vi "SendCmdToSkywireWaitToken.vi"(5 "Flush after? (y)":bool, 6 "Timeout (mSecs)":dbl=3500.0, 7 "Display err mess?":bool=TRUE, 8 "error in (no error)":errorcluster, 9 "Wait for token":string, 10 "Cmd String":string="AT+CSQ", 11 "VISA resource name":refnum<visa-resource-name>="COM30") -> (0 "error out":errorcluster, 1 "Response":string, 2 "timeout":bool, 3 "VISA resource name out":refnum<visa-resource-name>="COM30", 4 "Log resp":string)   [LabVIEW 2013]
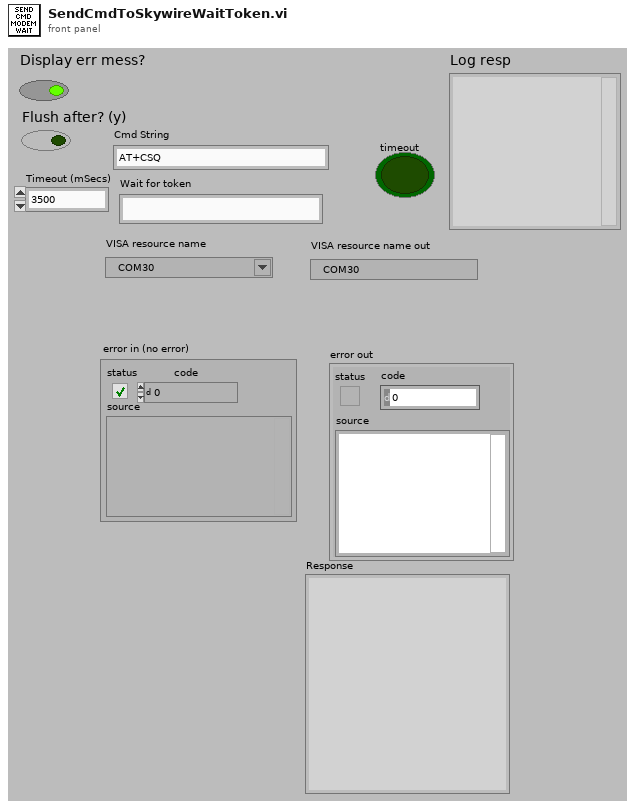
[diagram p1: front panel]
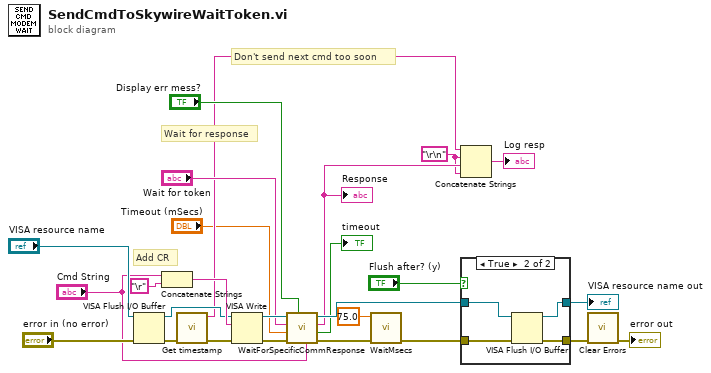
[diagram p0: block diagram]
diagram:
  w4 = "\r\n"
  # "Don't send next cmd too soon"
  # "Wait for response"
  # "Add CR"
  n1 = VISA Flush I/O Buffer(VISA resource name="VISA resource name", error in (no error)="error in (no error)") -> (VISA resource name out=w22:refnum<visa-resource-name>, error out=w8:errorcluster)  [unwired: 1 in]
  n2 = Concatenate Strings("Cmd String", "\r") -> (w25:string)
  n3 = call "Get timestamp.vi"("error in (no error)"=w8) -> ("error out"=w7:errorcluster, "Timestamp"=w6:string)  [unwired: 2 in, 7 out]
  n4 = VISA Write(VISA resource name=w22, write buffer=w25, error in (no error)=w7) -> (VISA resource name out=w17:refnum<visa-resource-name>, error out=w16:errorcluster)  [unwired: 1 out]
  n5 = call "WaitForSpecificCommResponse.vi"("CMD sent"="Cmd String", "Display err mess?"="Display err mess?", "error in (no error)"=w16, "Timeout (mSecs)"="Timeout (mSecs)", "Wait for"="Wait for token", "VISA Refnum in"=w17) -> ("error out"=w15:errorcluster, "timeout"=→"timeout":bool, "Response"=w5:string, "VISA Refnum out"=w14:refnum<visa-resource-name>)  [unwired: 1 in, 1 out]
  "Response" <- w5
  n6 = call "WaitMsecs.vi"("error in (no error)"=w15, "Wait Msecs"=75.0) -> ("error out"=w19:errorcluster)  [unwired: 9 in]
  n7 = Concatenate Strings(w6, w4, w5, w4) -> (→"Log resp":string)
  n8 = case shown="True" "Flush after? (y)" {
    tunnel: [w28 w32] -> w24
    tunnel: [w27 w31] -> w21
    tunnel: w19 -> [w28 w30]
    tunnel: w14 -> [w27 w29]
    frame False {
    }
    frame True {
      n9 = VISA Flush I/O Buffer(VISA resource name=w29, error in (no error)=w30) -> (VISA resource name out=w31:refnum<visa-resource-name>, error out=w32:errorcluster)  [unwired: 1 in]
    }
  }
  "VISA resource name out" <- w21
  n10 = call <vilib>:"Clear Errors.vi"("error in (no error)"=w24) -> ("error out"=→"error out":errorcluster)  [unwired: 6 in]
